vi "TP_FP_cal.vi"(7 "Target_order":path=path "C:/Users/Jaehong/Desktop/안전복지프로젝트/LabVIEW/RSVP_offline_onine/분석데이터/전선미_RSVP_Training_Test(LDA)/2014-08-29/ERP_Parameters_of_Target_prior.txt") -> (3 "TP+FP(%)":dbl)   [LabVIEW 2014]
uses:
  <vilib>/Utility/file.llb/Read From Spreadsheet File (I64).vi
panel:
  in  "ERP_발생_total":path=path "C:/Users/Jaehong/Desktop/안전복지프로젝트/LabVIEW/RSVP_offline_onine/분석데이터/전선미_RSVP_Training_Test(LDA)/2014-08-29/ERP_Parameters_of_Target_prior.txt"
  out "x*y":i32
  out "TP+FP":i16
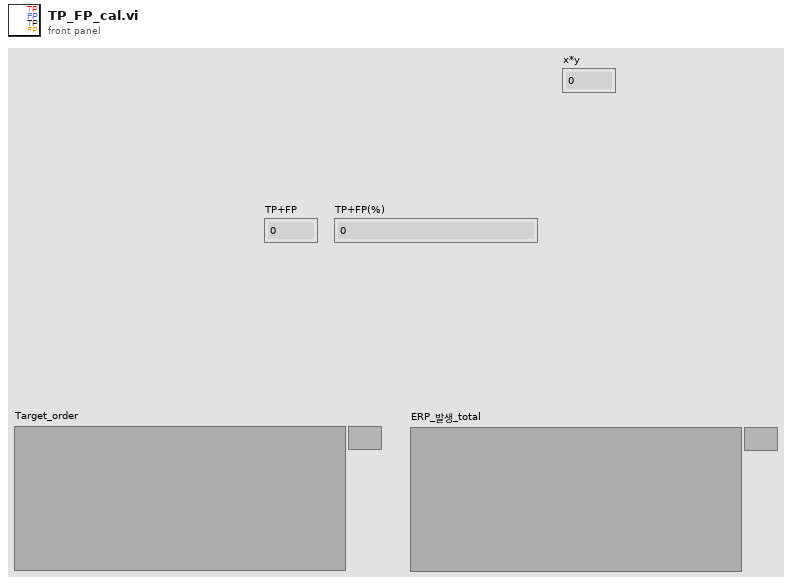
[diagram p1: front panel]
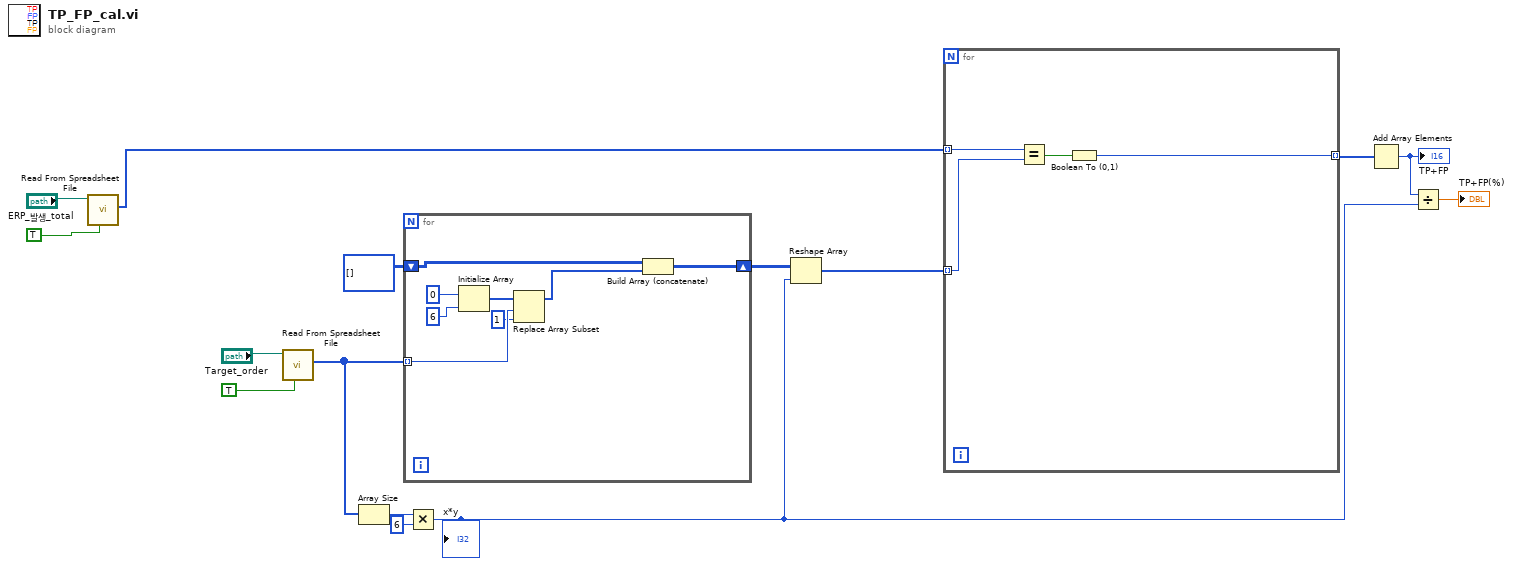
[diagram p0: block diagram]
diagram:
  n1 = call-poly <vilib>:"Read From Spreadsheet File.vi"("transpose (no:F)"=TRUE, "file path (dialog if empty)"="ERP_발생_total") -> ("first row"=w2:i64[])  [unwired: 5 in, 4 out]
  n2 = call-poly <vilib>:"Read From Spreadsheet File.vi"("transpose (no:F)"=TRUE, "file path (dialog if empty)"="Target_order") -> ("first row"=w11:i64[])  [unwired: 5 in, 4 out]
  n3 = Array Size(array=w11) -> (size(s)=w10:i32)
  n4 = for {
    tunnel: w11 -> [w20] mode=indexing
    shift-right: [w17] -> w12
    shift-left: i32[][] [] -> [w16]
    n5 = Initialize Array(0, 6) -> (w21:i32[])
    n6 = Replace Array Subset(array=w21, new element=1 ("new element/subarray"), index=w20) -> (w18:i32[])
    n7 = Build Array (concatenate)(w16, w18) -> (w17:i32[][])
  }
  n8 = Multiply(x=w10, y=6) -> (x*y=w5:i32)
  "x*y" <- w5
  n9 = Reshape Array(w12, w5) -> (w8:i32[])
  n10 = for {
    tunnel: w8 -> [w26] mode=indexing
    tunnel: w2 -> [w27] mode=indexing
    tunnel: [w24] -> w7 mode=indexing
    n11 = Equal?(x=w27, y=w26) -> (x = y?=w25:bool)
    n12 = Boolean To (0,1)(Boolean=w25) -> (0, 1=w24:i16)
  }
  n13 = Add Array Elements(numeric array=w7) -> (sum=w6:i16)
  "TP+FP" <- w6
  n14 = Divide(x=w6, y=w5) -> (x/y=→"TP+FP(%)":dbl)
